vi "Set Initialization Data - User.vi"(8 "error in":errorcluster, 11 "Manager Worker in":refnum<class "Manager Worker.lvclass">) -> (0 "error out":errorcluster, 3 "Manager Worker out":refnum<class "Manager Worker.lvclass">)   [LabVIEW 2018, in "Manager Worker.lvclass"]
doc: "Sets the initialization data of a statically linked subWorker."
uses:
  Manager Worker.lvclass
  User Worker/Initialization Data.ctl
  Manager Worker.lvclass/Manager Worker.ctl
  User Worker/User Worker.lvclass
  D:/Program Files (x86)/National Instruments/LabVIEW 2018/vi.lib/addons/_Workers/Library/Classes/Worker/Worker.lvclass
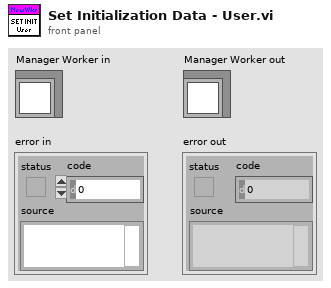
[diagram p1: front panel]
types:
  T1 = typedef "User Worker.lvclass/Initialization Data.ctl" = cluster{"String":string}
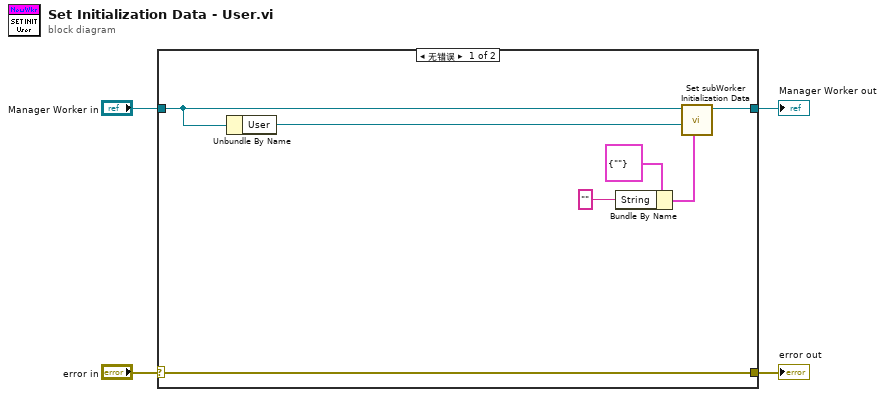
[diagram p0: block diagram]
diagram:
  n1 = case shown="无错误" "error in" {
    selector: "error in" -> [w11 w13]
    tunnel: [w11 w13] -> w3
    tunnel: [w9 w12] -> w2
    tunnel: "Manager Worker in" -> [w8 w12]
    frame No Error {
      n2 = Unbundle By Name(w8) -> ("User"=w10:refnum<class "User Worker.lvclass">)
      n3 = Bundle By Name(cluster=T1 {"String"=""} ("Initialization Data"), "String"="" ("Placeholder")) -> (w6:T1)
      n4 = call-dynamic "Set subWorker Initialization Data.vi"("Initialization Data"=w6, "subWorker"=w10, "Worker"=w8) -> ("Worker out"=w9:refnum<class "Manager Worker.lvclass">)  [unwired: 8 in]
    }
    frame Error {
    }
  }
  "error out" <- w3
  "Manager Worker out" <- w2
